vi "simple write to text.vi"(8 "error in":errorcluster, 10 "Background":i32[](array[numeric]), 11 "file path (use dialog)":path=path "C:/Users/BoasLab/Documents/Data/Alazar data/B-line/background/background.txt") -> (0 "error out":errorcluster)   [LabVIEW 2018]
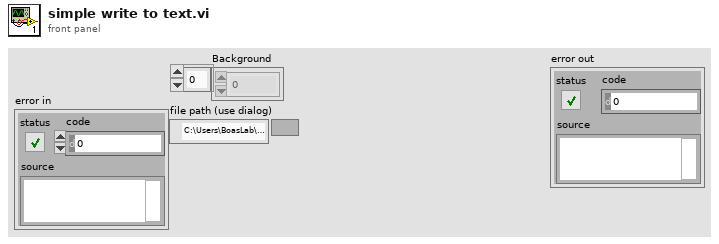
[diagram p1: front panel]
types:
  T1 = enum16{"open", "replace", "create", "open or create", "replace or create", "replace or create with confirmation"}
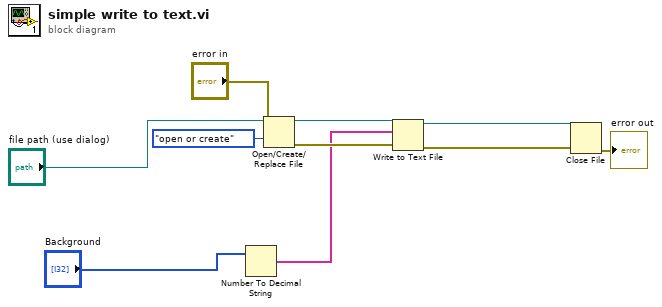
[diagram p0: block diagram]
diagram:
  n1 = Number To Decimal String(number="Background") -> (decimal integer string=w1:string[])  [unwired: 1 in]
  n2 = Open/Create/Replace File(file path (use dialog)="file path (use dialog)", error in="error in", operation (0:open)=T1."open or create") -> (refnum out=w5:refnum<file>, error out=w8:errorcluster)  [unwired: 3 in, 1 out]
  n3 = Write to Text File(file (use dialog)=w5, text=w1, error in=w8) -> (refnum out=w4:refnum<file>, error out=w7:errorcluster)  [unwired: 1 in, 1 out]
  n4 = Close File(refnum=w4, error in=w7) -> (error out=→"error out":errorcluster)  [unwired: 1 out]
